vi "Generate Timing Table.vi"(8 "error in (no error)":errorcluster, 11 "Performance Analyzer In":refnum<class "Execution Profiler Result View.lvclass">) -> (0 "error out":errorcluster, 2 "Timing List":string[](array[string]), 3 "Performance Analyzer Out":refnum<class "Execution Profiler Result View.lvclass">)   [LabVIEW 2020, in "Execution Profiler.lvlib" / "Execution Profiler Result View.lvclass"]
uses:
  Execution Profiler Result View/Execution Profiler Result View.lvclass
  Execution Profiler Result View/Execution Profiler Result View.lvclass/Execution Profiler Result View.ctl
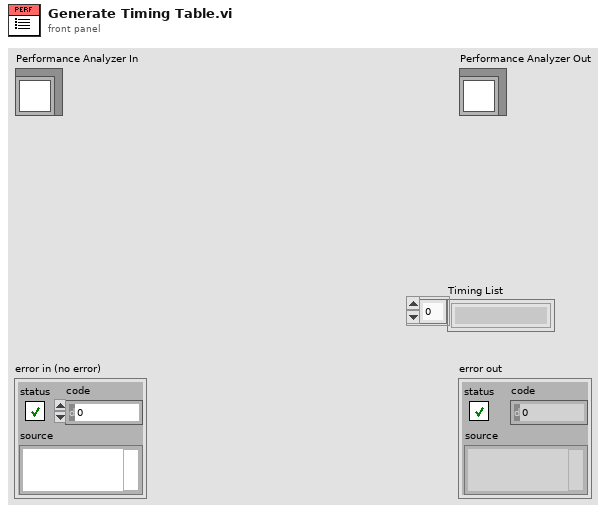
[diagram p1: front panel]
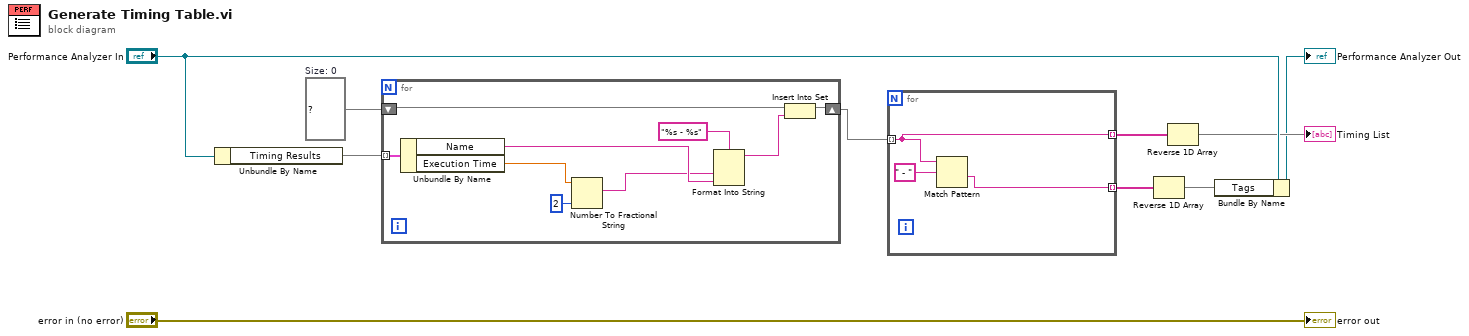
[diagram p0: block diagram]
diagram:
  w2 = set{string} {}  # Size: 0
  n1 = Unbundle By Name("Performance Analyzer In") -> ("Timing Results"=w8:map{string, dbl})
  n2 = for {
    tunnel: w8 -> [w19] mode=indexing
    shift-right: [w13] -> w1
    shift-left: w2 -> [w12]
    n3 = Unbundle By Name(w19) -> ("Name"=w15:string, "Execution Time"=w17:dbl)
    n4 = Number To Fractional String(number=w17, precision (6)=i16 2) -> (F-format string=w14:string)  [unwired: 2 in]
    n5 = Format Into String(format string="%s - %s", w14, w15) -> (resulting string=w11:string)  [unwired: 2 in, 1 out]
    n6 = Insert Into Set(10:w11, 11:w12) -> (3:w13:set{string})  [unwired: 1 out]
  }
  n7 = for {
    tunnel: w1 -> [w21] mode=indexing
    tunnel: [w21] -> w7 mode=indexing
    tunnel: [w20] -> w5 mode=indexing
    n8 = Match Pattern(string=w21, regular expression=" - " ("format string")) -> (after substring=w20:string)  [unwired: 1 in, 3 out]
  }
  n9 = Reverse 1D Array(array=w5) -> (reversed array=w3:string[])
  n10 = Reverse 1D Array(array=w7) -> (reversed array=→"Timing List":string[])
  n11 = Bundle By Name(cluster="Performance Analyzer In", "Tags"=w3) -> (→"Performance Analyzer Out":refnum<class "Execution Profiler Result View.lvclass">)
  "error out" <- "error in (no error)"
